vi "toString.vi"(8 "error in (no error)":errorcluster, 11 "IBaseObject in":refnum<class "IBaseObject.lvclass">) -> (0 "error out":errorcluster, 2 "string":string, 3 "IBaseObject out":refnum<class "IBaseObject.lvclass">)   [LabVIEW 2022 SP3, in "openDAQ.lvlib" / "IBaseObject.lvlib" / "IBaseObject.lvclass"]
uses:
  <instrlib>/openDAQ/Public/Classes/IBaseObject/IBaseObject.lvclass
  <instrlib>/openDAQ/Public/Classes/IBaseObject/IBaseObject.lvclass/IBaseObject.ctl
  <instrlib>/openDAQ/Public/Classes/IBaseObject/Accessor/Read reference.vi
  <instrlib>/openDAQ/Binaries/Windows/x86/copendaq32.dll
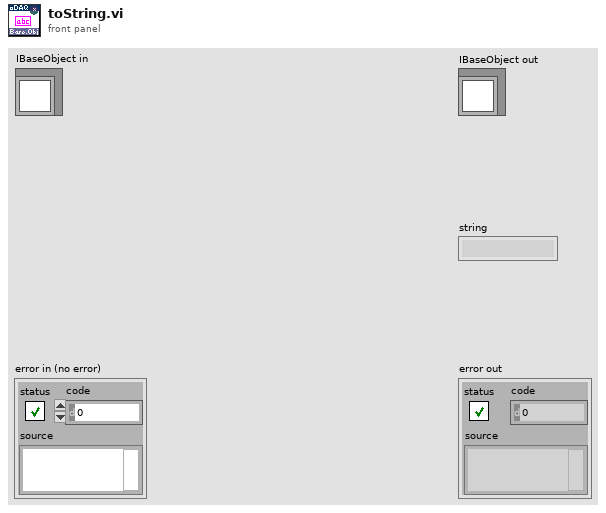
[diagram p1: front panel]
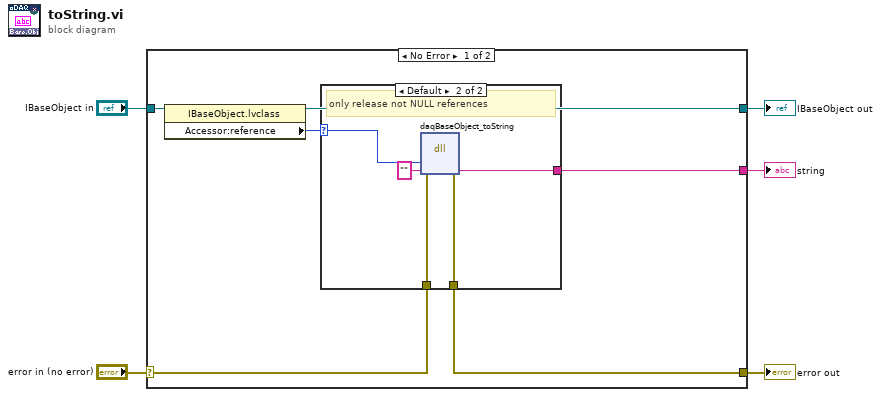
[diagram p0: block diagram]
diagram:
  n1 = case shown="No Error" "error in (no error)" {
    selector: "error in (no error)" -> [w11 w19]
    tunnel: [w10 w19] -> w4
    tunnel: "IBaseObject in" -> [w9 w18]
    tunnel: [w7 w18] -> w1
    tunnel: [w6 _] -> w2
    frame No Error {
      n2 = property class="IBaseObject.lvclass"(reference=w9) -> (reference out=w7:refnum<class "IBaseObject.lvclass">, "Accessor:reference"=w8:i64)  [unwired: 1 in, 1 out]
      n3 = case shown="Default" w8 {
        selector: w8 -> [_ w15]
        tunnel: w11 -> [w12 w17]
        tunnel: [w12 w16] -> w10
        tunnel: [_ w14] -> w6
        frame 0 {
        }
        frame Default {
          # "only release not NULL references"
          n4 = dll-call lib="C:/Program Files (x86)/National Instruments/LabVIEW 2022/instr.lib/openDAQ/Binaries/Windows/x86/copendaq*.*" fn="daqBaseObject_toString"(error in=w17, "baseObject"=w15, "string"="") -> (error out=w16:errorcluster, "string"=w14:string)  [unwired: 4 in, 1 out]
        }
      }
    }
    frame Error {
    }
  }
  "error out" <- w4
  "string" <- w2
  "IBaseObject out" <- w1
